vi "WF - Change Name and or Y vector.vi"(0 "wForm IN":waveform(dbl), 5 "error in (no error)":errorcluster, 6 "Attribute Option":T1, 7 "SigName Update":string, 9 "New Y Data":dbl[](array[numeric]) format="%#.6g") -> (14 "wForm OUT":waveform(dbl), 19 "error out":errorcluster)   [LabVIEW 2022 SP3, in "GSwFormDSP.lvclass"]
uses:
  GSwFormDSP.lvclass
  functions/Attribute Options.ctl
  functions/Attribute List.ctl
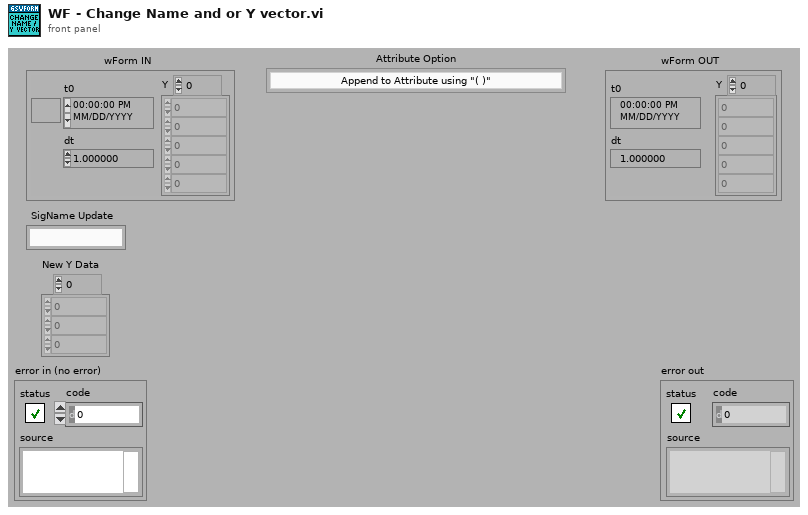
[diagram p1: front panel]
types:
  T1 = typedef "GSwFormDSP.lvclass/Attribute Options.ctl" = enum16{"Append to Attribute using \"( )\"", "Replace Attribute Value"}
  T2 = typedef "GSwFormDSP.lvclass/Attribute List.ctl" = string
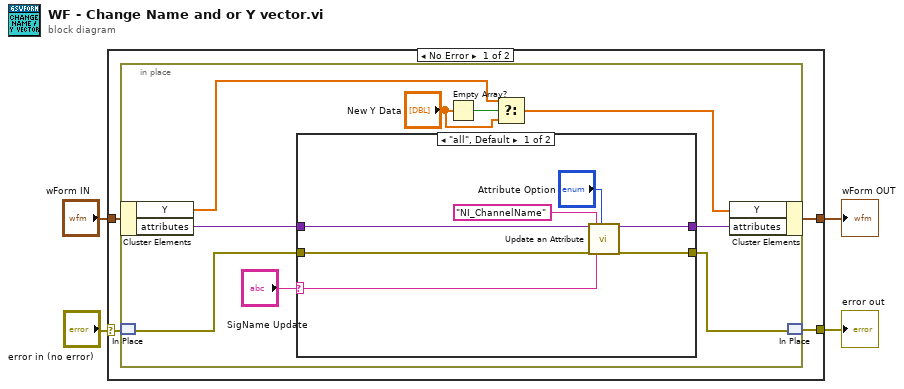
[diagram p0: block diagram]
diagram:
  n1 = case shown="No Error" "error in (no error)" {
    selector: "error in (no error)" -> [w7 w28]
    tunnel: [w5 w28] -> w3
    tunnel: [w6 w27] -> w1
    tunnel: "wForm IN" -> [w8 w27]
    frame No Error {
      n2 = in-place {
        n3 = in-place-cluster #1(w8) -> ("Y"=w11:dbl[], "attributes"=w15:variant)
        n4 = in-place-match #2(w7) -> (w13:errorcluster)
        n5 = case shown="\"all\", Default" "SigName Update" {
          selector: "SigName Update" -> [w18 _]
          tunnel: [w23 w26] -> w17
          tunnel: w15 -> [w20 w26]
          tunnel: w13 -> [w24 w25]
          tunnel: [w22 w25] -> w16
          frame "all", Default {
            n6 = call "Update an Attribute.vi"("attributes in"=w20, "error in (no error)"=w24, "Attribute List"=T2 "NI_ChannelName" ("wForm Attributes"), "Attribute Value"=w18, "Attribute Option"="Attribute Option") -> ("attributes out"=w23:variant, "error out"=w22:errorcluster)  [unwired: 13 in]
          }
          frame "" {
            # "Empty Signal name, so do nothing."
          }
        }
        n7 = Empty Array?(array="New Y Data") -> (empty?=w12:bool)
        n8 = Select(t=w11, s=w12, f="New Y Data") -> (s? t:f=w9:dbl[])
        n9 = in-place-cluster #1("Y"=w9, "attributes"=w17) -> (w6:waveform(dbl))
        n10 = in-place-match #2(w16) -> (w5:errorcluster)
      }
    }
    frame Error {
    }
  }
  "error out" <- w3
  "wForm OUT" <- w1
